vi "Get ListView Item Ref.vi"(8 "error in (no error)":errorcluster caption="错误输入（无错误）", 10 "index":i32, 11 "ListViewClass 输入":refnum<class "ListViewClass.lvclass"> caption="DNL_LabVIEW Object in") -> (0 "error out":errorcluster caption="错误输出", 2 "get_Item":refnum<k24>, 3 "ListViewClass 输出":refnum<class "ListViewClass.lvclass"> caption="DNL_LabVIEW Object out")   [LabVIEW 2012, in "ListViewClass.lvclass"]
uses:
  ListViewClass.lvclass
  System.Windows.Forms
  ListViewClass.lvclass/ListViewClass.ctl
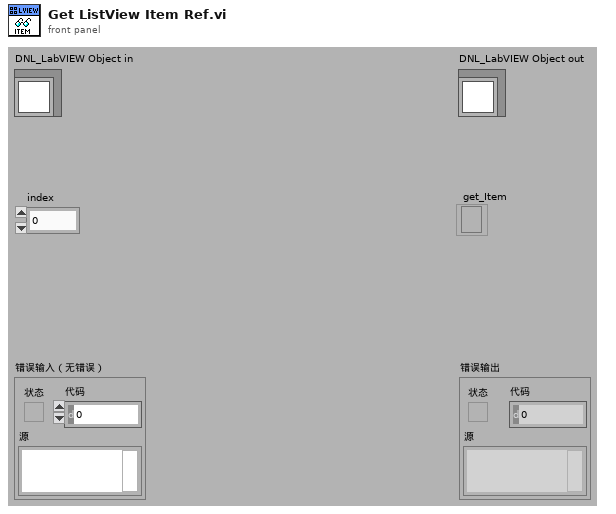
[diagram p1: front panel]
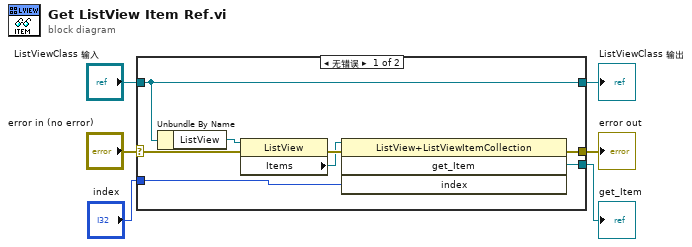
[diagram p0: block diagram]
diagram:
  n1 = case shown="无错误" "error in (no error)" {
    selector: "error in (no error)" -> [w8 w16]
    tunnel: [w7 w16] -> w5
    tunnel: [w14 w15] -> w3
    tunnel: "ListViewClass 输入" -> [w14 w15]
    tunnel: "index" -> [w11 _]
    tunnel: [w10 _] -> w1
    frame No Error {
      n2 = Unbundle By Name(w14) -> ("ListView"=w9:refnum<k24>)
      n3 = property class="ListView"(reference=w9, error in=w8) -> (error out=w13:errorcluster, "Items"=w12:refnum<k24>)  [unwired: 1 out]
      n4 = invoke class="ListView+ListViewItemCollection" method="get_Item"(reference=w12, error in=w13, "index"=w11) -> (error out=w7:errorcluster, "get_Item"=w10:refnum<k24>)  [unwired: 1 in, 2 out]
    }
    frame Error {
    }
  }
  "error out" <- w5
  "ListViewClass 输出" <- w3
  "get_Item" <- w1
